vi "Check Existing Configuration.vi"(8 "error in":errorcluster, 11 "Item Ref in":T1 format="%.0x") -> (0 "error out":errorcluster, 2 "Existing Configuration Exists":bool, 3 "Item Ref out":T1 format="%.0x")   [LabVIEW 2019, in "SEECD System Explorer.lvlib"]
uses:
  SEECD System Explorer.lvlib
  <vilib>/NI VeriStand/Custom Device API/Custom Device Item Ref.ctl
  Shared/Globals/Scan Engine GUIDs.vi
  <vilib>/NI VeriStand/Custom Device API/Custom Device API.lvlib
  Shared/SEECD Shared.lvlib
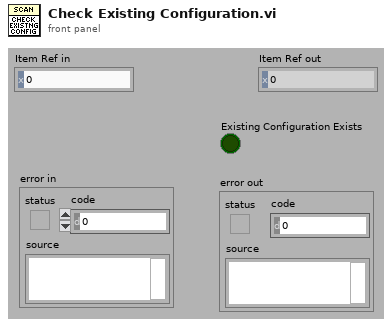
[diagram p1: front panel]
types:
  T1 = typedef "Custom Device API.lvlib/Custom Device Item Ref.ctl" = u64
  T2 = typedef "Custom Device API.lvlib/Custom Device Item Info.ctl" = cluster{"Name":string, "Is Channel":bool, "GUID":string, "Is Waveform":bool}
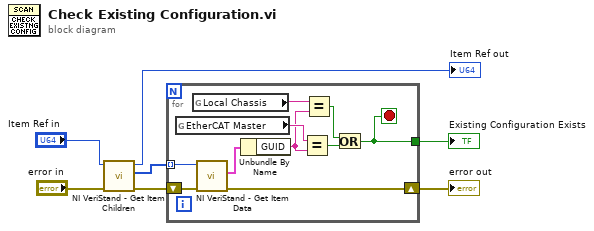
[diagram p0: block diagram]
diagram:
  n1 = call <vilib>:"NI VeriStand - Get Item Children.vi"("error in (no error)"="error in", "Item Ref in"="Item Ref in") -> ("error out"=w6:errorcluster, "Child Refs"=w7:T1[], "Item Ref out"=→"Item Ref out":T1)  [unwired: 6 in, 1 out]
  n2 = for {
    tunnel: w7 -> [w17] mode=indexing
    shift-right: [w9] -> w4
    shift-left: w6 -> [w16]
    tunnel: [w8] -> w1
    stop <- w8 stop-if-true
    n3 = global read "Scan Engine GUIDs.vi" "EtherCAT Master"() -> (w14:string)
    n4 = global read "Scan Engine GUIDs.vi" "Local Chassis"() -> (w13:string)
    n5 = call <vilib>:"NI VeriStand - Get Item Data.vi"("error in (no error)"=w16, "Item Ref in"=w17) -> ("error out"=w9:errorcluster, "Item Info"=w15:T2)  [unwired: 6 in, 2 out]
    n6 = Unbundle By Name(w15) -> ("GUID"=w12:string)
    n7 = Equal?(x=w14, y=w12) -> (x = y?=w10:bool)
    n8 = Equal?(x=w13, y=w12) -> (x = y?=w11:bool)
    n9 = Or(x=w11, y=w10) -> (x .or. y?=w8:bool)
  }
  "error out" <- w4
  "Existing Configuration Exists" <- w1
